vi "Graphik laufend.vi"(6 "Mittelwertdaten":sgl[][](array[numeric]), 7 "Numerisch":sgl, 9 "Komponenten Indices":i32[](array[numeric]), 10 "Zeitstempeln":timestamp[](array[timestamp]), 11 "Messdaten":sgl[][](array[numeric])) -> (2 "Refernz":waveform(sgl), 3 "Graph Array":waveform(dbl)[](array[waveform]))   [LabVIEW 2020, in "EPA 1065.lvlib" / "HovaCAL Interference verificaton.lvlib"]
uses:
  HovaCAL Interference verificaton.lvlib
  Seiten/FT-IR/FGV FT-IR Parameter.vi
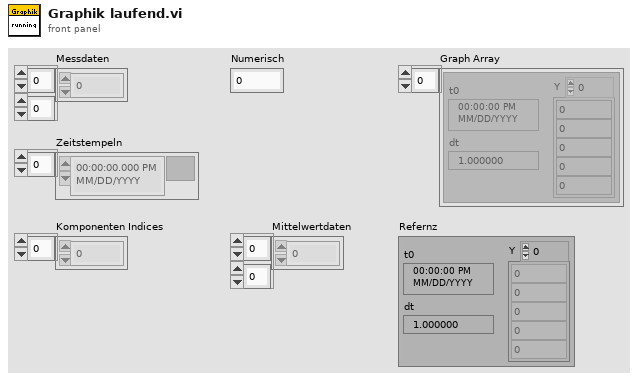
[diagram p1: front panel]
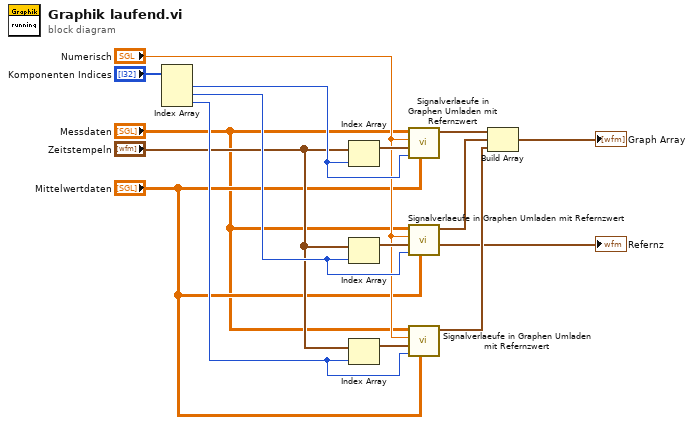
[diagram p0: block diagram]
diagram:
  n1 = Index Array(array="Komponenten Indices") -> (element #1=w14:i32, element #2=w9:i32, element #3=w8:i32)  [unwired: 3 in]
  n2 = Index Array(array="Zeitstempeln", index=w14) -> (element=w13:timestamp)
  n3 = Index Array(array="Zeitstempeln", index=w9) -> (element=w11:timestamp)
  n4 = Index Array(array="Zeitstempeln", index=w8) -> (element=w10:timestamp)
  n5 = call "Signalverlaeufe in Graphen Umladen mit Refernzwert.vi"("Mittelwertdaten"="Mittelwertdaten", "Gas-Auswahl"=w14, "t0"=w13, "Referenz in"="Numerisch", "Werte"="Messdaten") -> ("Waveform"=w16:waveform(dbl))  [unwired: 1 in, 5 out]
  n6 = call "Signalverlaeufe in Graphen Umladen mit Refernzwert.vi"("Mittelwertdaten"="Mittelwertdaten", "Gas-Auswahl"=w9, "t0"=w11, "Referenz in"="Numerisch", "Werte"="Messdaten") -> ("Refernz"=→"Refernz":waveform(sgl), "Waveform"=w4:waveform(dbl))  [unwired: 1 in, 4 out]
  n7 = call "Signalverlaeufe in Graphen Umladen mit Refernzwert.vi"("Mittelwertdaten"="Mittelwertdaten", "Gas-Auswahl"=w8, "t0"=w10, "Referenz in"="Numerisch", "Werte"="Messdaten") -> ("Waveform"=w3:waveform(dbl))  [unwired: 1 in, 5 out]
  n8 = Build Array(w16, w4, w3) -> (→"Graph Array":waveform(dbl)[])
